vi "Clear Task.vi"(8 "error in (no error)":errorcluster, 11 "DAQ Task in":refnum<class "DAQ Task.lvclass">) -> (0 "error out":errorcluster, 3 "DAQ Task out":refnum<class "DAQ Task.lvclass">)   [LabVIEW 2018, in "Data Acquisition.lvlib" / "DAQ Task.lvclass"]
uses:
  DAQ Task.lvclass
  DAQ Task.lvclass/DAQ Task.ctl
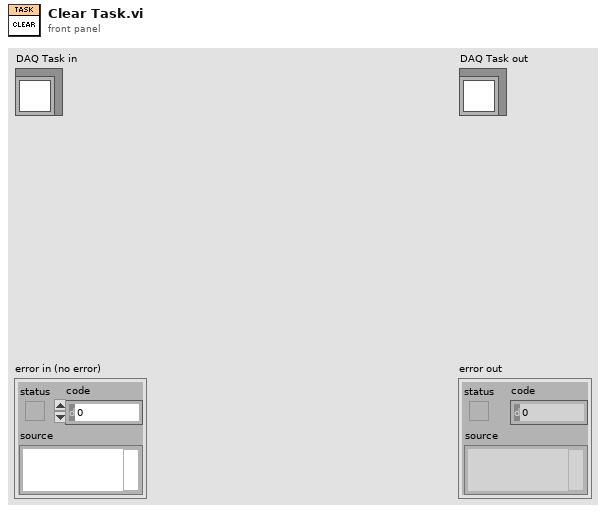
[diagram p1: front panel]
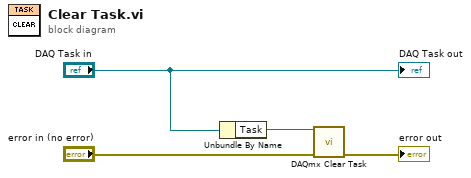
[diagram p0: block diagram]
diagram:
  n1 = Unbundle By Name("DAQ Task in") -> ("Task"=w1:refnum<k21>)
  n2 = call <vilib>:"DAQmx Clear Task.vi"("task in"=w1, "error in"="error in (no error)") -> ("error out"=→"error out":errorcluster)  [unwired: 13 in]
  "DAQ Task out" <- "DAQ Task in"
